vi "Tools_String Match String with Wildcard Pattern List.vi"(3 "case matching (sensitive)":T1=enum."system", 4 "string":string, 5 "pattern list":string[](array[string])=["lybraryn.llb/*", "memmon.llb/*"]) -> (0 "found substring":bool, 1 "match pattern":string, 2 "index":i32)   [LabVIEW 2012]
uses:
  Tools_String Case Matching.ctl
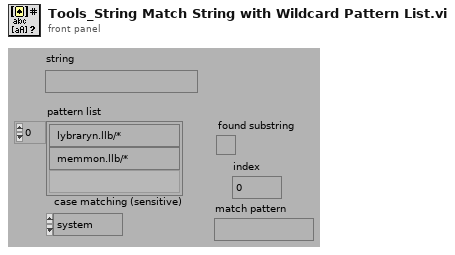
[diagram p1: front panel]
types:
  T1 = typedef "Tools_String Case Matching.ctl" = enum16{"a != A", "a == A", "system"}
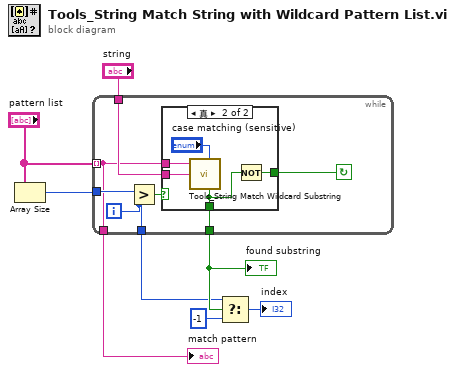
[diagram p0: block diagram]
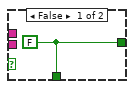
[diagram p2: hidden frame]
diagram:
  n1 = Array Size(array="pattern list") -> (size(s)=w6:i32)
  n2 = while {
    tunnel: [w9] -> w1
    tunnel: [w10] -> w3
    tunnel: [w12] -> w5
    tunnel: "string" -> [w14]
    tunnel: w6 -> [w15]
    tunnel: "pattern list" -> [w9] mode=indexing
    i -> [w10]
    stop <- w11 continue-if-true
    n3 = Greater?(x=w15, y=w10) -> (0:w13:bool)
    n4 = case shown="真" w13 {
      tunnel: w14 -> [_ w21]
      tunnel: w9 -> [_ w20]
      tunnel: [w16 w19] -> w12
      tunnel: [w16 w18] -> w11
      frame False {
        w16 = FALSE
      }
      frame True {
        n5 = call "Tools_String Match Wildcard Substring.vi"("case matching (sensitive)"="case matching (sensitive)", "string"=w21, "pattern with wildcards"=w20) -> ("found substring"=w19:bool)  [unwired: 1 in, 4 out]
        n6 = Not(x=w19) -> (.not. x?=w18:bool)
      }
    }
  }
  "found substring" <- w5
  "match pattern" <- w1
  n7 = Select(t=w3, s=w5, f=-1) -> (s? t:f=→"index":i32)
